vi "AuMT8852B Connection Time.vi"(8 "error in (no error)":errorcluster, 11 "VISA session":refnum<visa-resource-name>) -> (0 "error out":errorcluster, 2 "error code":i32, 3 "VISA session out":refnum<visa-resource-name>, 4 "Result":T1)   [LabVIEW 2017]
doc: "Anritsu MT8852B Bluetooth Tester\n\nDisplays the connection state, and if a connection is present, the time taken in milliseconds (ms) to make the connection when requested to connect to an EUT. On power on or before a connection has been made, the connection number displays as 0 (no connection) and is not followed by a time.\n\nOUTPUTS\nResult - displays the connection status and the time taken to connect if a connection exists."
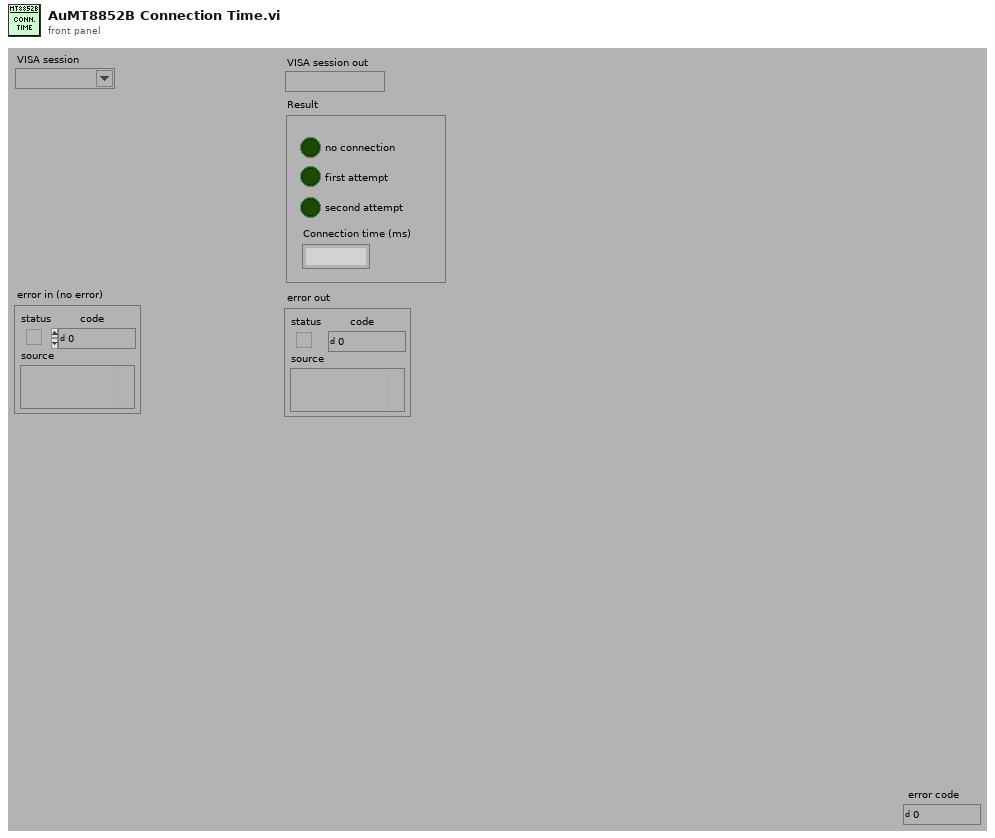
[diagram p1: front panel]
types:
  T1 = cluster{"no connection":bool, "first attempt":bool, "second attempt":bool, "Connection time (ms)":string}
  T2 = enum16{"Simulate", "Range check", "Cache", "Query instrument status"}
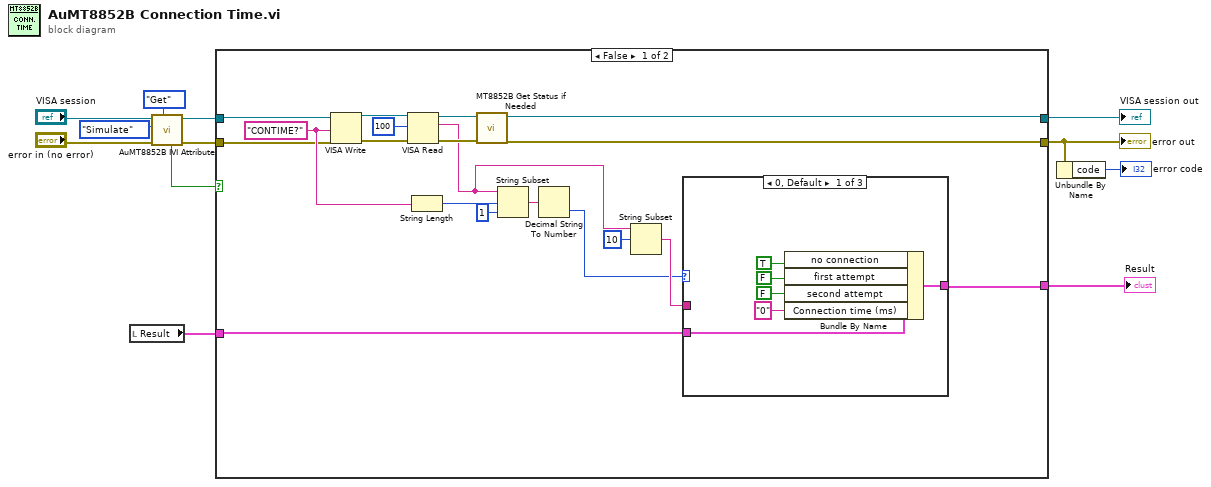
[diagram p0: block diagram]
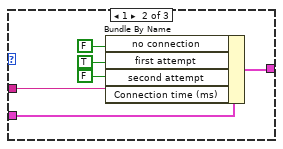
[diagram p2: hidden frame]
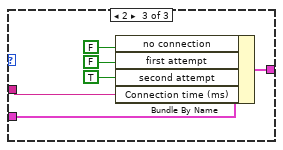
[diagram p3: hidden frame]
diagram:
  n1 = local read "Result"() -> (w1:T1)
  n2 = call <instrlib>:"AuMT8852B IVI Attribute.vi"("Set/Get (Set)"=enum16{"Set", "Get"}."Get", "error in (no error)"="error in (no error)", "Flag (Simulate)"=T2."Simulate", "VISA session"="VISA session") -> ("error out"=w8:errorcluster, "VISA session out"=w9:refnum<visa-resource-name>, "Value out"=w5:bool)  [unwired: 5 in]
  n3 = case shown="False" w5 {
    tunnel: [w15 w51] -> w3
    tunnel: [w14 w52] -> w10
    tunnel: w9 -> [w16 w52]
    tunnel: w8 -> [w17 w51]
    tunnel: [w18 w50] -> w2
    tunnel: w1 -> [w13 w50]
    frame False {
      w29 = "CONTIME?" ("write buffer (\"\")")
      n4 = VISA Write(VISA resource name=w16, write buffer=w29, error in (no error)=w17) -> (VISA resource name out=w28:refnum<visa-resource-name>, error out=w27:errorcluster)  [unwired: 1 out]
      n5 = VISA Read(VISA resource name=w28, byte count=u32 100 ("byte count (0)"), error in (no error)=w27) -> (VISA resource name out=w30:refnum<visa-resource-name>, read buffer=w25:string, error out=w31:errorcluster)  [unwired: 1 out]
      n6 = String Length(string=w29) -> (length=w19:i32)
      n7 = call <instrlib>:"MT8852B Get Status if Needed.vi"("error in (no error)"=w31, "VISA session"=w30) -> ("error out"=w15:errorcluster, "VISA session out"=w14:refnum<visa-resource-name>)  [unwired: 8 in]
      n8 = String Subset(string=w25, offset (0)=w19, length (rest)=1 ("length (rest)")) -> (substring=w21:string)
      n9 = Decimal String To Number(string=w21) -> (number=w22:i32)  [unwired: 2 in, 1 out]
      n10 = String Subset(string=w25, offset (0)=10) -> (substring=w24:string)  [unwired: 1 in]
      n11 = case shown="0, Default" w22 {
        tunnel: [w37 w39 w44] -> w18
        tunnel: w13 -> [w36 w40 w45]
        tunnel: w24 -> [_ w38 w46]
        frame 0, Default {
          n12 = Bundle By Name(cluster=w36, "no connection"=TRUE, "first attempt"=FALSE, "second attempt"=FALSE ("no connection"), "Connection time (ms)"="0") -> (w37:T1)
        }
        frame 1 {
          n13 = Bundle By Name(cluster=w40, "no connection"=FALSE, "first attempt"=TRUE, "second attempt"=FALSE ("no connection"), "Connection time (ms)"=w38) -> (w39:T1)
        }
        frame 2 {
          n14 = Bundle By Name(cluster=w45, "no connection"=FALSE, "first attempt"=FALSE, "second attempt"=TRUE ("no connection"), "Connection time (ms)"=w46) -> (w44:T1)
        }
      }
    }
    frame True {
    }
  }
  "error out" <- w3
  "VISA session out" <- w10
  "Result" <- w2
  n15 = Unbundle By Name(w3) -> ("code"=→"error code":i32)
